vi "queryPose.vi"(0 "连接ID":refnum<k5>) -> (1 "连接ID输出":refnum<k5>, 2 "x":dbl, 3 "vx":dbl, 4 "y":dbl, 5 "z":dbl, 6 "vy":dbl, 7 "vz":dbl)   [LabVIEW 2017]
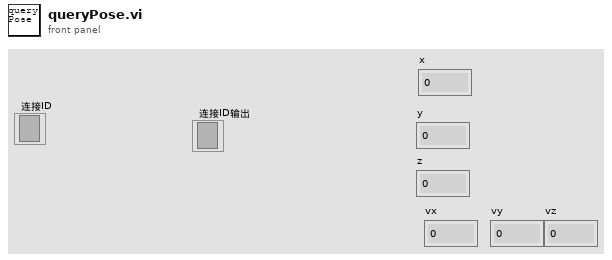
[diagram p1: front panel]
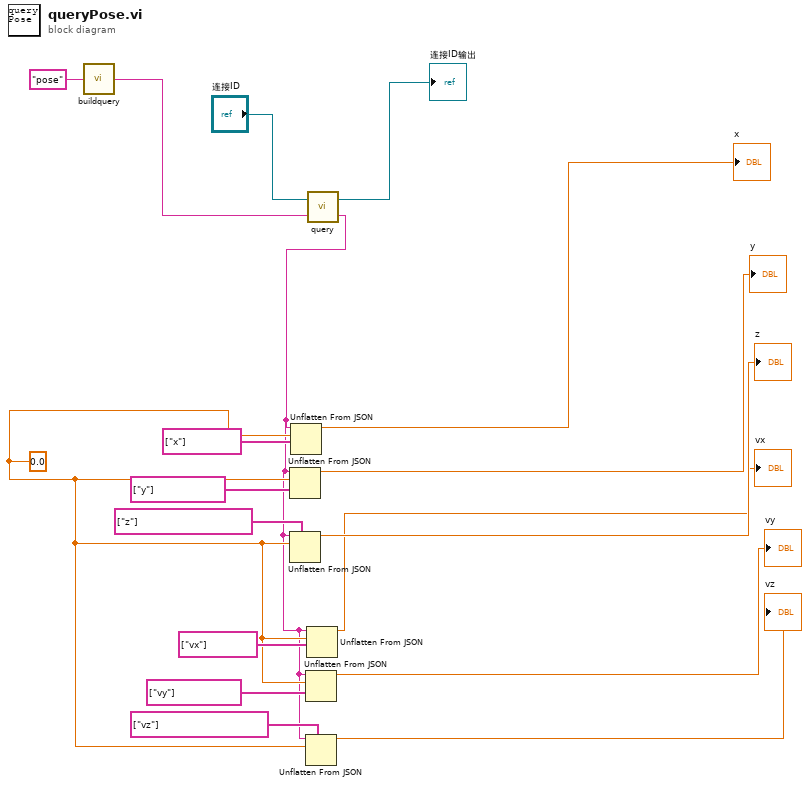
[diagram p0: block diagram]
diagram:
  w8 = 0.0 ("z home speed 2")
  n1 = call "buildquery.vi"("String"="pose") -> ("JSON字符串"=w15:string)
  n2 = call "query.vi"("数据输入"=w15, "连接ID"="连接ID") -> ("数据输出"=w7:string, "连接ID输出"=→"连接ID输出":refnum<k5>)
  n3 = Unflatten From JSON(path=string[] ["y"] ("路径"), JSON string=w7, type and defaults=w8) -> (value=→"y":dbl)  [unwired: 4 in, 1 out]
  n4 = Unflatten From JSON(path=string[] ["z"] ("路径"), JSON string=w7, type and defaults=w8) -> (value=→"z":dbl)  [unwired: 4 in, 1 out]
  n5 = Unflatten From JSON(path=string[] ["x"] ("路径"), JSON string=w7, type and defaults=w8) -> (value=→"x":dbl)  [unwired: 4 in, 1 out]
  n6 = Unflatten From JSON(path=string[] ["vy"] ("路径"), JSON string=w7, type and defaults=w8) -> (value=→"vy":dbl)  [unwired: 4 in, 1 out]
  n7 = Unflatten From JSON(path=string[] ["vz"] ("路径"), JSON string=w7, type and defaults=w8) -> (value=→"vz":dbl)  [unwired: 4 in, 1 out]
  n8 = Unflatten From JSON(path=string[] ["vx"] ("路径"), JSON string=w7, type and defaults=w8) -> (value=→"vx":dbl)  [unwired: 4 in, 1 out]
